vi "AlliGator Set Image Display Range.vi"(3 "Display Image Control Refnum":T3, 5 "Image Histogram":refnum<vi>, 8 "Error In":errorcluster, 9 "Displayed Image?":T1, 10 "Displayed Image":T2, 11 "Image to Display":T2) -> (0 "Error Out":errorcluster, 1 "Palette Display Range":cluster{"Min Value":dbl, "Max Value":dbl}={"Min Value"=nan, "Max Value"=nan}, 2 "Image Display Range":cluster{"Min Value":dbl, "Max Value":dbl}={"Min Value"=nan, "Max Value"=nan}, 4 "CPU (s)":dbl)   [LabVIEW 2021, in "AlliGator Source Image.lvlib"]
doc: "Handles Source Image display range using the Histogram."
uses:
  AlliGator Source Image.lvlib
  Image/Image Control Refnum.ctl
  <vilib>/vision/Image Controls.llb/IMAQ Image.ctl
  AlliGator Displayed Image.ctl
  AlliGator Settings List.ctl
  Variant/Variant to Data/Variant to Boolean.vi
  <vilib>/vision/NI_Vision_Development_Module.lvlib
  AlliGator Settings.lvlib
  Variant/Variant to Data/Variant to Data.lvlib
  Image/Image.lvlib
panel:
  # "see the AlliGator License on the block diagram (Ctrl+E or Window:Show Block Diagram)"
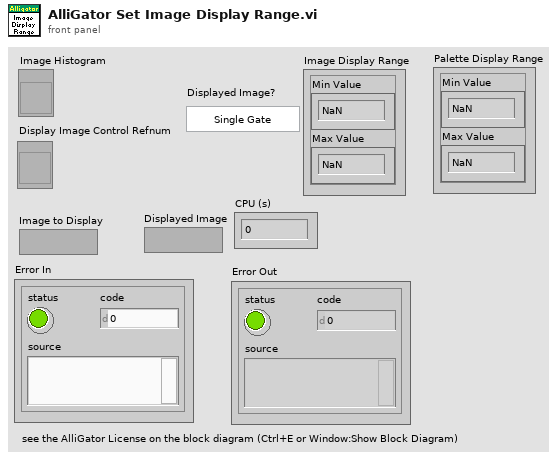
[diagram p1: front panel]
types:
  T1 = typedef "AlliGator Source Image.lvlib/AlliGator Displayed Image.ctl" = enum16{"Single Gate", "Sum of All Gates", "Max of All Gates", "Min of All Gates", "-", "White Ligth Image", "Mask Image"}
  T2 = typedef "IMAQ Image.ctl" = refnum<image>
  T3 = typedef "Image.lvlib/Image Control Refnum.ctl" = refnum<vi>
  T4 = typedef "AlliGator Settings.lvlib/AlliGator Settings List.ctl" = enum16{"GUI:Visible Settings Tab", "GUI:Last Run Version", "Source Image:Use Image Histogram for Contrast", "Source Image:Low Count Pixels Rejection Options", "Source Image:High Count Pixels Rejection Options", "Source Image:Use Image Brightness", "Source Image:Blend Overlay with Image Background", "Source Image:Use Fixed ROI Diameter", "Source Image:ROI Diameter", "Source Image:ROI Center Color", "Source Image:Peak Threshold", "Source Image:Intensity Threshold", "Source Image:Image Binning Options", "Source Image:Image Smoothing Options", "Source Image:Image Histogram Active", "Source Image:Invert Binary Mask", "Source Image:Hot Pixel Removal", "Source Image:Overlay Analyzed ROI Center", "Source Image:Auto-Adjust Contrast", "Source Image:Histogram Lower Percentile", "Source Image:Histogram Upper Percentile", "Source Image:Save Source Image", "Source Image:Scale Bar Options", "Source Image:Image Resolution (Pixel Size)", "Source Image:Flatfield Correction", "Data Information:Gate Width", "Data Information:Nanotime Gate Separation", "Data Information:Macrotime Gate Separation", "Data Information:Gate Step", "Data Information:# Gates", "Data Information:Gate Image Exposure", "Data Information:Gate Image Integration", "Data Information:Gates to Skip", "Data Information:Gates to Keep", "Data Information:Define Gates to", "Data Information:Channel Name", "Data Information:Available Channel Names", "Data Information:Channel Arithmetic", "Data Information:Background File Subtraction", "Data Information:Background File", "Data Information:Background Scaling Factor", "Data Information:Background Pile-up Correction", "Data Information:Background Pixel Well Capacity", "Data Information:Laser Period", "Data Information:SYNC Period", "Data Information:Pile-up Correction", "Data Information:Pixel Well Capacity", "Data Information:Dataset Scaling Factor", "Fluorescence Decay_Decay Pre-Processing:Reverse Gates", "Fluorescence Decay_Decay Pre-Processing:Verbose Decay Pre-Processing", "Fluorescence Decay_Decay Pre-Processing:Use Decay Pre-Processing", "Fluorescence Decay_Decay Pre-Processing:Background Subtraction", "Fluorescence Decay_Decay Pre-Processing:Background Definition Range", "Fluorescence Decay_Decay Pre-Processing:Baseline Subtraction Method", "Fluorescence Decay_Decay Pre-Processing:Operations Order", "Fluorescence Decay_Decay Pre-Processing:Smoothing Parameter", "Fluorescence Decay_Decay Pre-Processing:Shift Decay", "Fluorescence Decay_Decay Pre-Processing:Decay Shift Parameters", "Fluorescence Decay_Decay Pre-Processing:Fold Decay", "Fluorescence Decay_Decay Pre-Processing:# Folds", "Fluorescence Decay_Decay Pre-Processing:1-Normalize Decay", "Fluorescence Decay_Decay Pre-Processing:[0-1]-Normalize Decay", "Fluorescence Decay_Decay Pre-Processing:Smoothen Decay", "Fluorescence Decay_Decay Pre-Processing:Extrapolate Decay", "Fluorescence Decay_Decay Pre-Processing:Use Periodicity", "Fluorescence Decay_Decay Pre-Processing:Use Cursors", "Fluorescence Decay_Decay Pre-Processing:Tail Fraction", "Fluorescence Decay_Decay Pre-Processing:Head Fraction", "Fluorescence Decay_Decay Pre-Processing:Additional Points", "Fluorescence Decay_Decay Pre-Processing:Straighten Decay", "Fluorescence Decay_Decay Pre-Processing:Constant Background", "Fluorescence Decay_Decay Pre-Processing:Pixel-Normalize Decay", "Fluorescence Decay_Advanced Analysis:Extract IRF instead of Decay", "Fluorescence Decay_Advanced Analysis:IRF Extraction Options", "Fluorescence Decay_Advanced Analysis:IRF Optimization Options", "Fluorescence Decay_Advanced Analysis:Square Pulse Options", "Fluorescence Decay_Advanced Analysis:IRF Order", "Fluorescence Decay_Advanced Analysis:IRF Time Constants", "Fluorescence Decay_Advanced Analysis:Wavelet Analysis Options", "Fluorescence Decay_Advanced Analysis:Average Lifetime Options", "Fluorescence Decay_Fit Options:Fit Options", "Fluorescence Decay_Fit Options:Use Legacy Fitting Approach", "Fluorescence Decay_Fit Options:Use Data Information Laser Period", "Fluorescence Decay_Fit Parameters:Displayed Fit Parameters", "Fluorescence Decay_Fit Parameters:Fit Parameter Constraints", "Fluorescence Decay_Fit Parameters:Export Tabulated Results", "Fluorescence Decay_Fit Parameters:MLE Baseline Offset Type", "Fluorescence Decay_Fit Parameters:MLE Baseline Offset", "Fluorescence Decay_Fit Parameters:Guess Parameter Names", "Fluorescence Decay_Fit Parameters:Guess Parameter Values", "Fluorescence Decay_Fit Parameters:Guess Parameters Options", "Fluorescence Decay_Styles:Show Last Decay Only", "Fluorescence Decay_Styles:Decay Graph Color Array", "Fluorescence Decay:Decay Graph Active", "Fluorescence Decay Statistics:Min Peak Value", "Fluorescence Decay Statistics:Reject Low Decay Peak Pixels", "Fluorescence Decay Statistics:Reject High Decay Peak Pixels", "Fluorescence Decay Statistics:Max Peak Value", "Time Traces:Use File Timestamp", "Time Traces:Time Step", "Time Traces:Use Intensity Correction File", "Time Traces:Intensity Correction File", "Phasor Plot:Phasor Plot Smoothing Options", "Phasor Plot:Phasor Plot Size", "Phasor Plot:Phasor Plot Graphics Options", "Phasor Plot:Cumulative Phasor Plot", "Phasor Plot:Use Phasor Brightness", "Phasor Plot:Blend Overlay with Phasor Background", "Phasor Plot:Save Phasor Plot", "Phasor Plot:Show References", "Phasor Plot:Phasor Ratio Decay Range", "Phasor Plot:Exponential Fading", "Phasor Plot:Phasor Ratio Reference Colors", "Phasor Plot:Reference Radius", "Phasor Plot:Show Color Map Vertices", "Phasor Plot:Phasor Plot Active", "Phasor Plot:Phasor Ratio Color Map Type", "Phasor Plot:Phasor Ratio Color Map", "Phasor Plot:Phasor Ratio Display Range", "Phasor Plot:Selected Image ROI(s)", "Phasor Plot:All Image ROIs", "Phasor Plot:Selected Phasor Plot ROI(s)", "Phasor Plot:All Phasor Plot ROIs", "Phasor Plot:Phasor Ratio Color-Coded Quantity", "Phasor Plot:Store Phasor Harmonics", "Phasor Plot:Draw Reference Segment", "Phasor Plot:User-Defined Quantity", "Phasor Graph:Phasor Frequency", "Phasor Graph:Phasor Ratio Type", "Phasor Graph:Pixel-level Phasor Computation", "Phasor Graph:Save Phasor Graph", "Phasor Graph:Phasor Graph Active", "Phasor Graph:Phasor SDV Options", "Phasor Calibration:Use Backup Calibration if needed", "Phasor Graph:Define Shortest Lifetime as", "Phasor Calibration:Backup Calibration Type", "Phasor Calibration:Calibration Type", "Phasor Calibration:Calibration Lifetime", "Phasor Calibration:Calibration Map Algorithm", "Single-Exponential Phasor Locus (SEPL):Gate Parameters", "Single-Exponential Phasor Locus (SEPL):User-defined Gate", "Single-Exponential Phasor Locus (SEPL):User-defined IRF", "Single-Exponential Phasor Locus (SEPL):Phasor Parameters", "Single-Exponential Phasor Locus (SEPL):Decay & IRF Parameters", "Single-Exponential Phasor Locus (SEPL):Display Parameters", "Lifetime Analysis:Decay Analysis Parameters", "Lifetime Analysis:Lifetime Map Active", "Plugins:Python Settings", "Miscellaneous:Verbose Mode", "Miscellaneous:Beep after Script", "Miscellaneous:Saved Image File Format", "Miscellaneous:Exported Gate Image Settings", "Miscellaneous:Include Loading in Timing", "Miscellaneous:Verbose Settings Mode", "Miscellaneous:Histogram Options", "Miscellaneous:Beep on Error", "Miscellaneous:# Logical Processors Used", "Miscellaneous:ROI Description Max Characters", "Miscellaneous:Verbose Error Mode", "Miscellaneous:Transparent Mask Color"}
  T5 = cluster{"histogram":u32[], "Minimal Value":sgl, "Maximal Value":sgl, "Starting Value":sgl, "Interval Width":sgl, "Mean Value":sgl, "Standard  Variation":sgl, "Area (pixels)":i32}
  T6 = typedef "Image Type" = u32
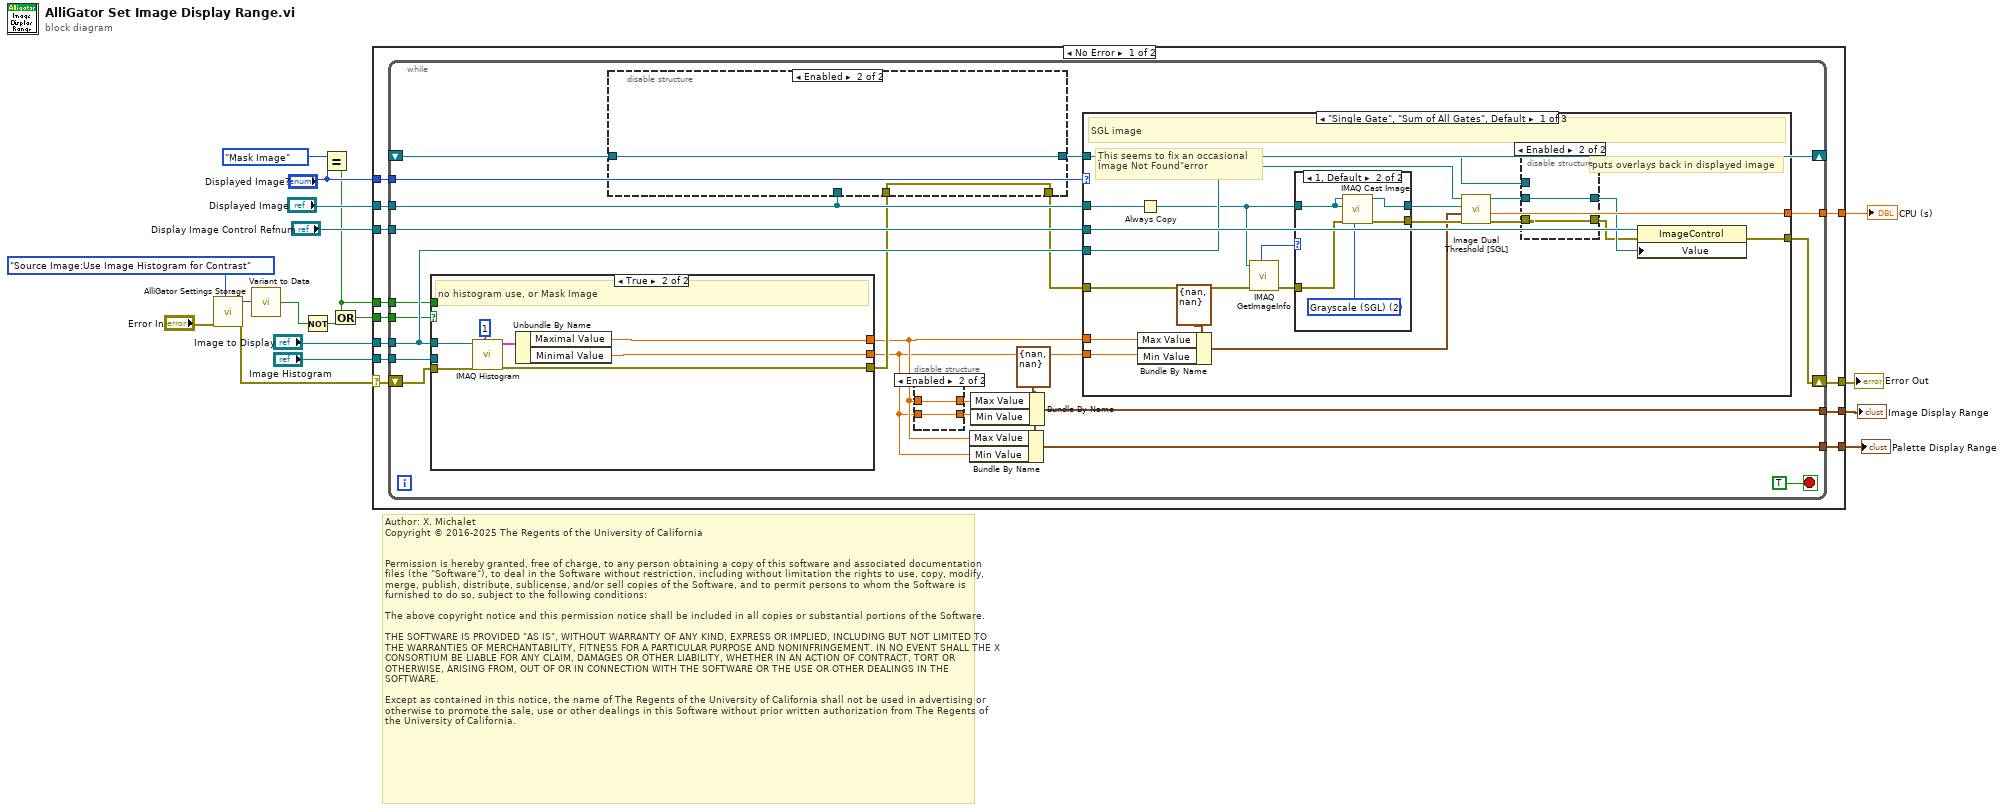
[diagram p0: block diagram]
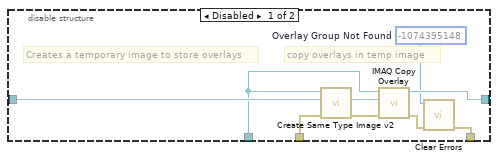
[diagram p2: hidden frame]
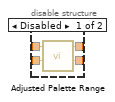
[diagram p3: hidden frame]
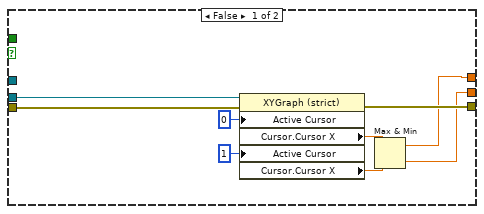
[diagram p4: hidden frame]
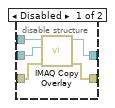
[diagram p5: hidden frame]
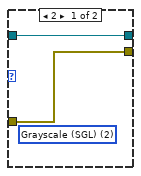
[diagram p6: hidden frame]
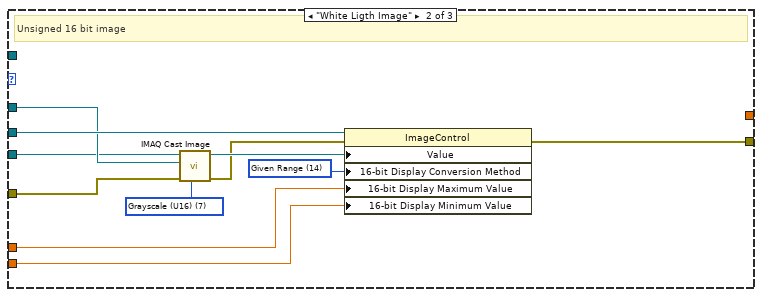
[diagram p7: hidden frame]
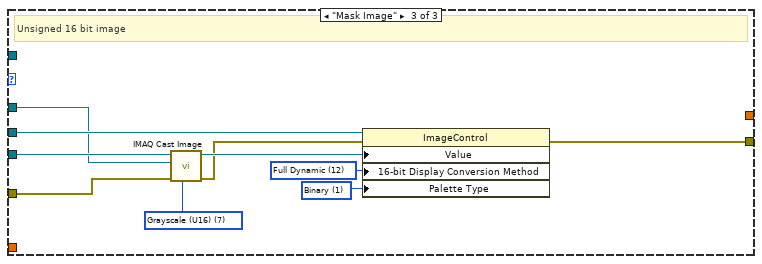
[diagram p8: hidden frame]
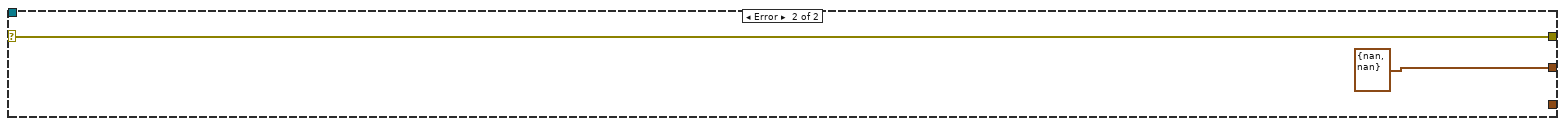
[diagram p9: hidden frame]
diagram:
  # "Author: X. Michalet\nCopyright © 2016-2025 The Regents of the University of California\n \n\nPermission is hereby granted, free of charge, to any person obtaining a copy of this software and associated documentation files (the \"Software\"), to deal in the Software without restriction, including without limitation the rights to use, copy, modify, merge, publish, distribute, sublicense, and/or sell copies of the Software, and to permit persons to whom the Software is furnished to do so, subject to the following conditions:\n\nThe above copyright notice and this permission notice shall be included in all copies or substantial portions of the Software.\n\nTHE SOFTWARE IS PROVIDED \"AS IS\", WITHOUT WARRANTY OF ANY KIND, EXPRESS OR IMPLIED, INCLUDING BUT NOT LIMITED TO THE WARRANTIES OF MERCHANTABILITY, FITNESS FOR A PARTICULAR PURPOSE AND NONINFRINGEMENT. IN NO EVENT SHALL THE X CONSORTIUM BE LIABLE FOR ANY CLAIM, DAMAGES OR OTHER LIABILITY, WHETHER IN AN ACTION OF CONTRACT, TORT OR OTHERWISE, ARISING FROM, OUT OF OR IN CONNECTION WITH THE SOFTWARE OR THE USE OR OTHER DEALINGS IN THE SOFTWARE.\n\nExcept as contained in this notice, the name of The Regents of the University of California shall not be used in advertising or otherwise to promote the sale, use or other dealings in this Software without prior written authorization from The Regents of the University of California."
  n1 = call "AlliGator Settings Storage.vi"("AlliGator Settings List"=AlliGator_Settings_List."Source Image:Use Image Histogram for Contrast", "Error In"="Error In") -> ("Error Out"=w3:errorcluster, "Variant Data out"=w6:variant)  [unwired: 8 in]
  n2 = call-poly "Variant to Data.vi"("Variant"=w6) -> ("Value"=w5:bool)  [unwired: 8 in]
  n3 = Not(x=w5) -> (.not. x?=w10:bool)
  n4 = Equal?(x=AlliGator_Displayed_Image."Mask Image" ("Displayed Image?"), y="Displayed Image?") -> (x = y?=w8:bool)
  n5 = Or(x=w8, y=w10) -> (x .or. y?=w9:bool)
  n6 = case shown="No Error" w3 {
    selector: w3 -> [w29 w142]
    tunnel: "Image Histogram" -> [w30 _]
    tunnel: "Display Image Control Refnum" -> [w28 _]
    tunnel: [w27 w142] -> w16
    tunnel: "Displayed Image" -> [w21 _]
    tunnel: [w20 cluster{"Min Value":dbl, "Max Value":dbl} {"Min Value"=nan, "Max Value"=nan} ("Image Display Range")] -> w14
    tunnel: "Image to Display" -> [w26 _]
    tunnel: "Displayed Image?" -> [w25 _]
    tunnel: w9 -> [w24 _]
    tunnel: w8 -> [w23 _]
    tunnel: [w22 _] -> w2
    tunnel: [w19 _] -> w1
    frame No Error {
      n7 = while {
        tunnel: w30 -> [w52]
        tunnel: w28 -> [w50]
        tunnel: w26 -> [w48]
        tunnel: w25 -> [w47]
        tunnel: w24 -> [w46]
        tunnel: w23 -> [w45]
        tunnel: [w44] -> w22
        tunnel: w21 -> [w41]
        shift-right: [w49] -> w27
        shift-left: w29 -> [w51]
        shift-right: [w40] -> _
        shift-left: _ -> [w42]
        tunnel: [w36] -> w20
        tunnel: [w32] -> w19
        stop <- TRUE stop-if-true
        w35 = cluster{"Min Value":dbl, "Max Value":dbl} {"Min Value"=nan, "Max Value"=nan} ("Image Display Range")
        n8 = case shown="True" w46 {
          tunnel: w52 -> [w78 _]
          tunnel: w51 -> [w75 w84]
          tunnel: [w72 w81] -> w39
          tunnel: [w71 w83] -> w34
          tunnel: [w70 w82] -> w33
          tunnel: w48 -> [_ w85]
          tunnel: w45 -> [_ _]
          frame False {
            n9 = property class="XYGraph (strict)"(reference=w78, error in=w75, "Active Cursor"=u32 0, "Active Cursor"=u32 1) -> (error out=w72:errorcluster, "Cursor.Cursor X"=w74:dbl, "Cursor.Cursor X"=w73:dbl)  [unwired: 1 out]
            n10 = Max & Min(x=w74, y=w73) -> (max(x,y)=w71:dbl, min(x,y)=w70:dbl)
          }
          frame True {
            # "no histogram use, or Mask Image"
            n11 = call "IMAQ Histogram"("Number of Classes"=1, "error in (no error)"=w84, "Image"=w85) -> ("error out"=w81:errorcluster, "Histogram Report"=w79:T5)  [unwired: 7 in]
            n12 = Unbundle By Name(w79) -> ("Maximal Value"=w83:sgl, "Minimal Value"=w82:sgl)
          }
        }
        n13 = disable-structure shown="Enabled" {
          disable-tunnel: w42 -> [w61 w63]
          disable-tunnel: w41 -> [w58 _]
          disable-tunnel: [w57 w63] -> w40
          disable-tunnel: w39 -> [w56 w62]
          disable-tunnel: [w53 w62] -> w31
          frame Disabled {
            w54 = -1074395148  # Overlay Group Not Found
            # "copy overlays in temp image"
            # "Creates a temporary image to store overlays"
            n14 = call "Create Same Type Image v2.vi"("error in (no error)"=w56, "Image Dst"=w61, "Image Src"=w58) -> ("error out"=w60:errorcluster, "Image Dst"=w59:T2)  [unwired: 6 in, 1 out]
            n15 = call "IMAQ Copy Overlay"("error in (no error)"=w60, "Image Dst"=w59, "Image Src"=w58) -> ("error out"=w55:errorcluster, "Image Dst Out"=w57:T2)  [unwired: 7 in]
            n16 = call <vilib>:"Clear Errors.vi"("error in (no error)"=w55, "specific error code to clear (0: all)"=w54) -> ("error out"=w53:errorcluster)  [unwired: 4 in, 1 out]
          }
          frame Enabled {
          }
        }
        n17 = disable-structure shown="Enabled" {
          disable-tunnel: [w67 w69] -> w38
          disable-tunnel: [w66 w68] -> w37
          disable-tunnel: w33 -> [w65 w69]
          disable-tunnel: w34 -> [w64 w68]
          frame Disabled {
            n18 = call "Adjusted Palette Range.vi"("Image Min"=w65, "Image Max"=w64) -> ("Palette Range Min"=w67:sgl, "Palette Range Max"=w66:sgl)  [unwired: 7 in, 1 out]
          }
          frame Enabled {
          }
        }
        n19 = Bundle By Name(cluster=w35, "Max Value"=w34, "Min Value"=w33) -> (w32:cluster{"Min Value":dbl, "Max Value":dbl})
        n20 = Bundle By Name(cluster=w35, "Max Value"=w37, "Min Value"=w38) -> (w36:cluster{"Min Value":dbl, "Max Value":dbl})
        n21 = case shown="\"Single Gate\", \"Sum of All Gates\", Default" w47 {
          tunnel: w34 -> [w90 w121 _]
          tunnel: w33 -> [w89 w120 _]
          tunnel: [w104 w123 w133] -> w49
          tunnel: w50 -> [w105 w130 w140]
          tunnel: w31 -> [w101 w125 w136]
          tunnel: w48 -> [w102 w128 w139]
          tunnel: w41 -> [w96 w129 w137]
          tunnel: [w98 _ _] -> w44
          tunnel: w40 -> [w94 _ _]
          frame "Single Gate", "Sum of All Gates", Default {
            # "This seems to fix an occasional Ïmage Not Found\"error"
            # "puts overlays back in displayed image"
            # "SGL image"
            n22 = Always Copy(1:w96) -> (0:w86:T2)
            n23 = Bundle By Name(cluster=cluster{"Min Value":dbl, "Max Value":dbl} {"Min Value"=nan, "Max Value"=nan} ("Image Display Range"), "Max Value"=w90, "Min Value"=w89) -> (w87:cluster{"Min Value":dbl, "Max Value":dbl})
            n24 = call "IMAQ GetImageInfo"("error in (no error)"=w101, "Image"=w86) -> ("error out"=w100:errorcluster, "Image Type"=w99:T6)  [unwired: 2 in, 6 out]
            n25 = case shown="1, Default" w99 {
              tunnel: [w113 w119] -> w103
              tunnel: [w114 w118] -> w97
              tunnel: w100 -> [w113 w117]
              tunnel: w86 -> [w114 w116]
              frame 2 {
                (unwired) T6 2 items=["Grayscale (U8)", "Grayscale (I16)", "Grayscale (SGL)", "Complex (CSG)", "RGB (U32)", "HSL (U32)", "RGB (U64)", "Grayscale (U16)"] ("Image Type")
              }
              frame 1, Default {
                w115 = T6 2 items=["Grayscale (U8)", "Grayscale (I16)", "Grayscale (SGL)", "Complex (CSG)", "RGB (U32)", "HSL (U32)", "RGB (U64)", "Grayscale (U16)"] ("Image Type")
                n26 = call "IMAQ Cast Image"("Image Type"=w115, "error in (no error)"=w117, "Image Dst"=w116, "Image Src"=w116) -> ("error out"=w119:errorcluster, "Image Dst Out"=w118:T2)  [unwired: 6 in]
              }
            }
            n27 = call "Image Dual Threshold [SGL].vi"("error in (no error)"=w103, "Range"=w87, "Image Dst"=w97, "Image Src"=w102) -> ("error out"=w92:errorcluster, "CPU (s)"=w98:dbl, "Image Dst Out"=w95:T2)  [unwired: 5 in]
            n28 = disable-structure shown="Enabled" {
              disable-tunnel: w95 -> [w110 w112]
              disable-tunnel: w94 -> [w109 _]
              disable-tunnel: [w108 w112] -> w93
              disable-tunnel: w92 -> [w107 w111]
              disable-tunnel: [w106 w111] -> w91
              frame Disabled {
                n29 = call "IMAQ Copy Overlay"("error in (no error)"=w107, "Image Dst"=w110, "Image Src"=w109) -> ("error out"=w106:errorcluster, "Image Dst Out"=w108:T2)  [unwired: 7 in]
              }
              frame Enabled {
              }
            }
            n30 = property class="ImageControl"(reference=w105, error in=w91, "Value"=w93) -> (error out=w104:errorcluster)  [unwired: 1 out]
          }
          frame "White Ligth Image" {
            w124 = T6 7 items=["Grayscale (U8)", "Grayscale (I16)", "Grayscale (SGL)", "Complex (CSG)", "RGB (U32)", "HSL (U32)", "RGB (U64)", "Grayscale (U16)"] ("Image Type")
            w122 = u32 14 items=["Default"=10, "Most Significant Bits"=11, "Full Dynamic"=12, "Downshift"=13, "Given Range"=14, "90% Dynamic"=15, "Given Percent Range"=16] ("16-bit Display Mapping:Conversion Method")
            # "Unsigned 16 bit image"
            n31 = call "IMAQ Cast Image"("Image Type"=w124, "error in (no error)"=w125, "Image Dst"=w129, "Image Src"=w128) -> ("error out"=w126:errorcluster, "Image Dst Out"=w127:T2)  [unwired: 6 in]
            n32 = property class="ImageControl"(reference=w130, error in=w126, "Value"=w127, "16-bit Display Conversion Method"=w122, "16-bit Display Maximum Value"=w121, "16-bit Display Minimum Value"=w120) -> (error out=w123:errorcluster)  [unwired: 1 out]
          }
          frame "Mask Image" {
            w132 = u32 12 items=["Default"=10, "Most Significant Bits"=11, "Full Dynamic"=12, "Downshift"=13, "Given Range"=14, "90% Dynamic"=15, "Given Percent Range"=16] ("16-bit Display Mapping:Conversion Method")
            w134 = T6 7 items=["Grayscale (U8)", "Grayscale (I16)", "Grayscale (SGL)", "Complex (CSG)", "RGB (U32)", "HSL (U32)", "RGB (U64)", "Grayscale (U16)"] ("Image Type")
            w131 = u32 1 items=["Grayscale", "Binary", "Gradient", "Rainbow", "Temperature", "User Defined", "Binary 16 Bit", "Gradient 16 Bit", "Rainbow 16 Bit", "Temperature 16 Bit", "User Defined 16 Bit"] ("Palette:Palette Type")
            # "Unsigned 16 bit image"
            n33 = call "IMAQ Cast Image"("Image Type"=w134, "error in (no error)"=w136, "Image Dst"=w137, "Image Src"=w139) -> ("error out"=w135:errorcluster, "Image Dst Out"=w138:T2)  [unwired: 6 in]
            n34 = property class="ImageControl"(reference=w140, error in=w135, "Value"=w138, "16-bit Display Conversion Method"=w132, "Palette Type"=w131) -> (error out=w133:errorcluster)  [unwired: 1 out]
          }
        }
      }
    }
    frame Error {
    }
  }
  "Error Out" <- w16
  "Image Display Range" <- w14
  "CPU (s)" <- w2
  "Palette Display Range" <- w1
